vi "Test Project Produces only one Suite.vi"(8 "error in (no error)":errorcluster, 11 "Test Case In":refnum<class "Test FInder Test.lvclass">) -> (0 "error out":errorcluster, 3 "Test Case Out":refnum<class "Test FInder Test.lvclass">)   [LabVIEW 2020, in "Test FInder Test.lvclass"]
uses:
  Test FInder Test.lvclass
  C:/Program Files (x86)/National Instruments/LabVIEW 2020/vi.lib/Astemes/LUnit/Test Case.lvclass
  Result/Type.ctl
  <vilib>/Astemes/LUnit/Test Case.lvclass/Test Case.ctl
  4ee1ff36-f2a2-4d81-80da-2416f687ba87.vi
  <vilib>/Astemes/LUnit/Palette/Pass.vi
  <vilib>/Astemes/LUnit/Palette/Fail.vi
  <vilib>/Astemes/LUnit/Compare Variants.vi
  <vilib>/Astemes/LUnit/Describe Comparison.vi
  <vilib>/Astemes/LUnit/Set Assertion Type.vi
  <vilib>/Astemes/LUnit/Add test result.vi
  <vilib>/Astemes/LUnit/Variant to string.vi
  <vilib>/Astemes/LUnit/LUnit Record Assertion Result.vi
  <vilib>/Astemes/LUnit/LUnit Aggregate Assertion Results.vi
  <vilib>/Astemes/LUnit/Method Result/LUnit Merge Status.vi
  <vilib>/Astemes/LUnit/LUnit Concatenate result strings.vi
  <vilib>/Utility/Data Type/Get Type Information.vi
  <vilib>/Utility/LVClass/Get LV Class Name.vi
  LUnit Test Suite/LUnit Test Suite V2.lvclass
  Test Finder/Test Finder V2.lvclass
  Result/Result.lvlib
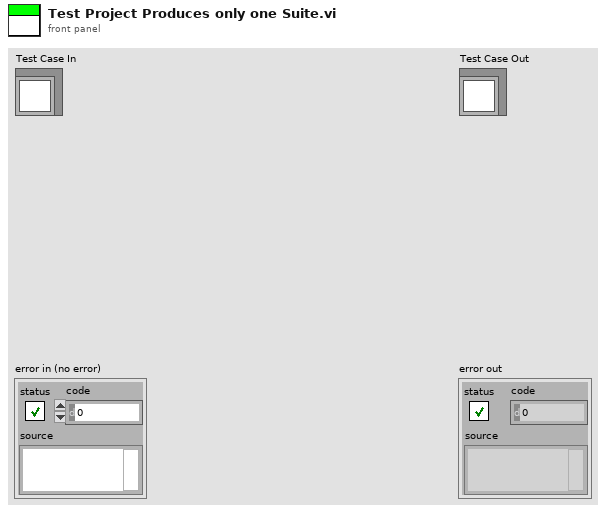
[diagram p1: front panel]
types:
  T1 = typedef "Result.lvlib/Result.ctl" = cluster{"Name":string, "Message":string, "Description":string, "Status":T2, "Result Type":T3, "Execution Time":dbl}
  T2 = typedef "Result.lvlib/Status.ctl" = enum16{"", "Passed", "Failed", "Error", "Skipped", "Setup Error", "Broken", "Teardown Error"}
  T3 = typedef "Result.lvlib/Type.ctl" = enum16{"Method", "Case", "Suite", "Pass", "Fail", "Skip", "Pass if", "Fail if", "Pass if Error", "Fail if Error", "Pass if Equal", "Fail if Equal"}
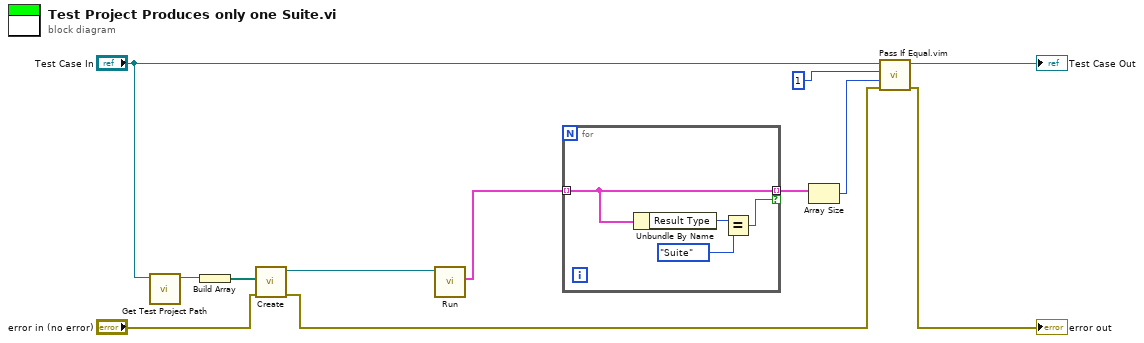
[diagram p0: block diagram]
diagram:
  n1 = call "Get Test Project Path.vi"("LUnit Test Suite Tests in"="Test Case In") -> ("appended path"=w9:path)  [unwired: 10 in]
  n2 = Build Array(w9) -> (w8:path[])
  n3 = call "Create.vi"("error in (no error)"="error in (no error)", "File Paths"=w8) -> ("error out"=w10:errorcluster, "LUnit Test Suite V2.lvclass"=w7:refnum<class "LUnit Test Suite V2.lvclass">)  [unwired: 8 in]
  n4 = call-dynamic "Run.vi"("Run in"=w7) -> ("Results"=w3:T1[])  [unwired: 9 in, 1 out]
  n5 = for {
    tunnel: w3 -> [w14] mode=indexing
    tunnel: [w14] -> w4 mode=indexing if=w13
    n6 = Unbundle By Name(w14) -> ("Result Type"=w16:T3)
    n7 = Equal?(x=w16, y=Type."Suite") -> (x = y?=w13:bool)
  }
  n8 = Array Size(array=w4) -> (size(s)=w2:i32)
  n9 = call "Pass If Equal.vim"("error in (no error)"=w10, "Actual"=w2, "Expected"=1 ("size(s)"), "LUnit Test Case In"="Test Case In") -> ("error out"=→"error out":errorcluster, "LUnit Test Case Out"=→"Test Case Out":refnum<class "Test FInder Test.lvclass">)  [unwired: 6 in]
